vi "Write configuration to device.vi"(2 "error in (no error)":errorcluster, 3 "FP ref in":T1) -> (0 "error out":errorcluster)   [LabVIEW 2020]
uses:
  Typedefs/Front Panel Object References.ctl
  Typedefs/SDCP - Serial Port Control - Commands.ctl
  Typedefs/SDCP - Standard Message Frames FGV - Commands.ctl
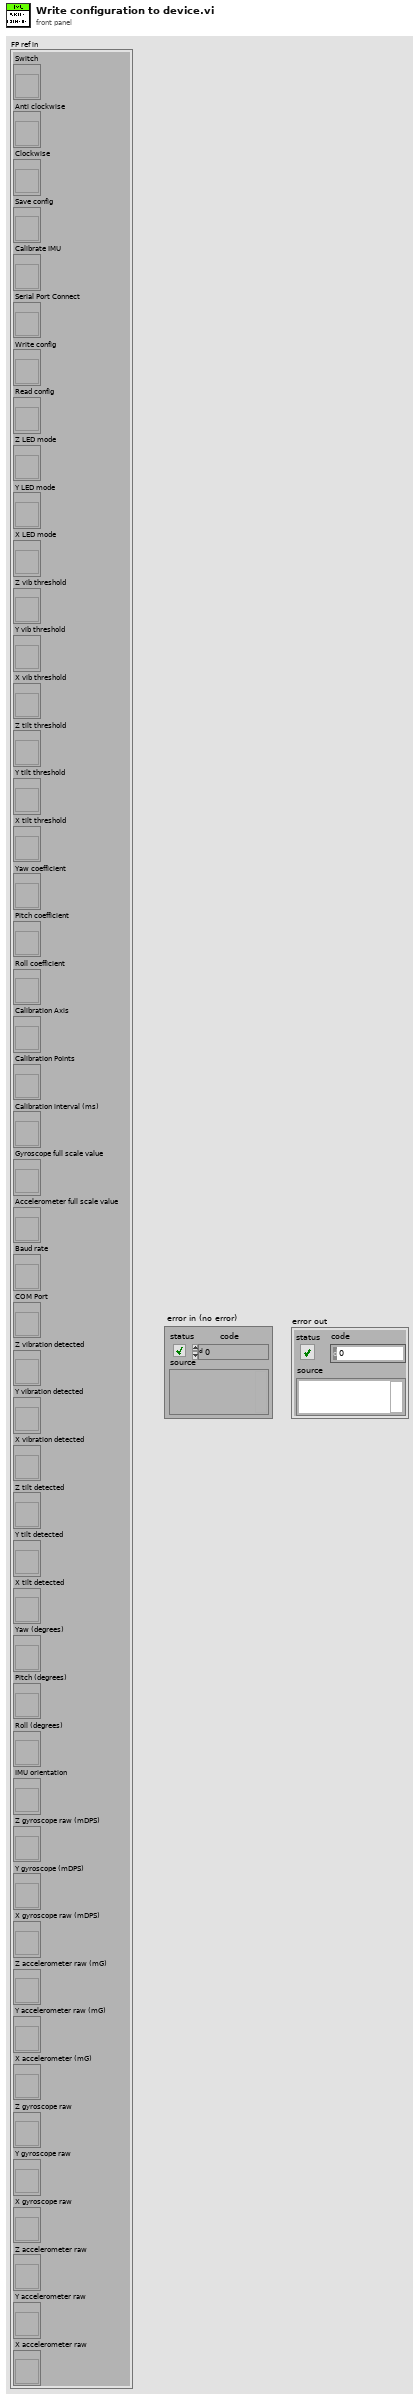
[diagram p1: front panel]
types:
  T1 = typedef "Front Panel Object References.ctl" = cluster{"Switch":refnum<vi>, "Anti clockwise":refnum<vi>, "Clockwise":refnum<vi>, "Save config":refnum<vi>, "Calibrate IMU":refnum<vi>, "Serial Port Connect":refnum<vi>, "Write config":refnum<vi>, "Read config":refnum<vi>, "Z LED mode":refnum<vi>, "Y LED mode":refnum<vi>, "X LED mode":refnum<vi>, "Z vib threshold":refnum<vi>, "Y vib threshold":refnum<vi>, "X vib threshold":refnum<vi>, "Z tilt threshold":refnum<vi>, "Y tilt threshold":refnum<vi>, "X tilt threshold":refnum<vi>, "Yaw coefficient":refnum<vi>, "Pitch coefficient":refnum<vi>, "Roll coefficient":refnum<vi>, "Calibration Axis":refnum<vi>, "Calibration Points":refnum<vi>, "Calibration interval (ms)":refnum<vi>, "Gyroscope full scale value":refnum<vi>, "Accelerometer full scale value":refnum<vi>, "Baud rate":refnum<vi>, "COM Port":refnum<vi>, "Z vibration detected":refnum<vi>, "Y vibration detected":refnum<vi>, "X vibration detected":refnum<vi>, "Z tilt detected":refnum<vi>, "Y tilt detected":refnum<vi>, "X tilt detected":refnum<vi>, "Yaw (degrees)":refnum<vi>, "Pitch (degrees)":refnum<vi>, "Roll (degrees)":refnum<vi>, "IMU orientation":refnum<vi>, "Z gyroscope raw (mDPS)":refnum<vi>, "Y gyroscope (mDPS)":refnum<vi>, "X gyroscope raw (mDPS)":refnum<vi>, "Z accelerometer raw (mG)":refnum<vi>, "Y accelerometer raw (mG)":refnum<vi>, "X accelerometer (mG)":refnum<vi>, "Z gyroscope raw":refnum<vi>, "Y gyroscope raw":refnum<vi>, "X gyroscope raw":refnum<vi>, "Z accelerometer raw":refnum<vi>, "Y accelerometer raw":refnum<vi>, "X accelerometer raw":refnum<vi>}
  T2 = typedef "SDCP - Serial Port Control - Commands.ctl" = enum16{"Open", "Read", "Write", "Get instance", "Close"}
  T3 = enum16{"X positive", "X neagtive", "Y positive", "Y negative", "Z positive", "Z negative"}
  T4 = typedef "LED mode.ctl" = enum16{"Tilt detection", "Vibration detection", "Accelerometer magnitude", "Gyroscope magnitude", "GPIO test", "PWM test"}
  T5 = typedef "SDCP - Standard Message Frames FGV - Commands.ctl" = enum16{"Reset", "Read", "Write", "Set Priority"}
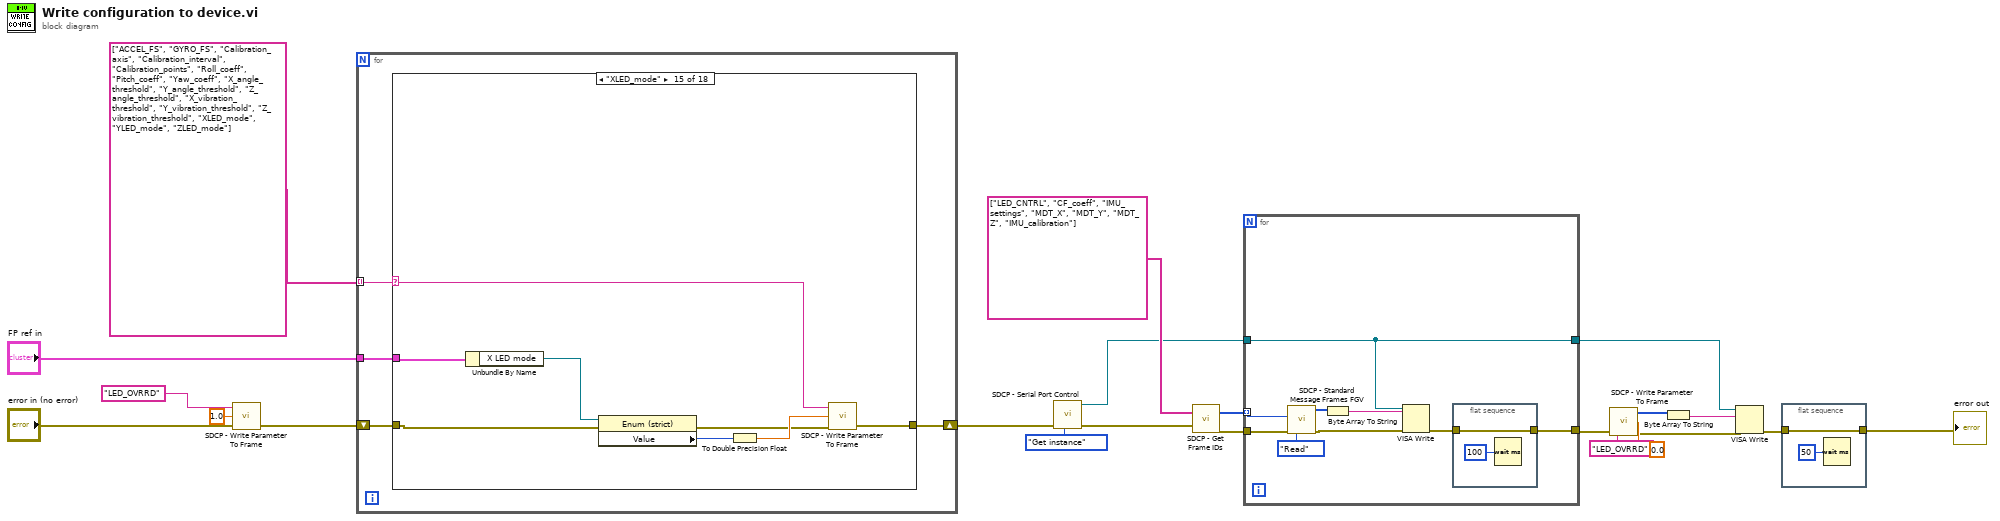
[diagram p0: block diagram]
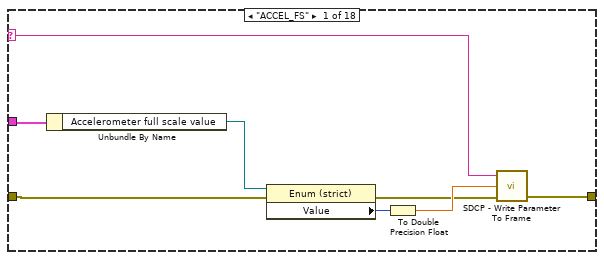
[diagram p2: hidden frame]
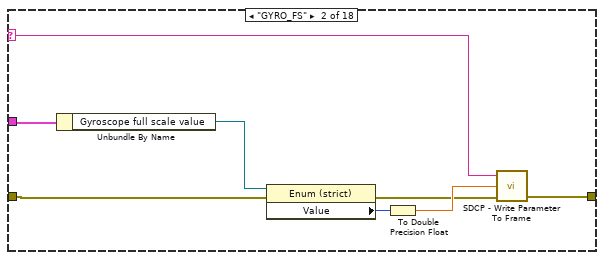
[diagram p3: hidden frame]
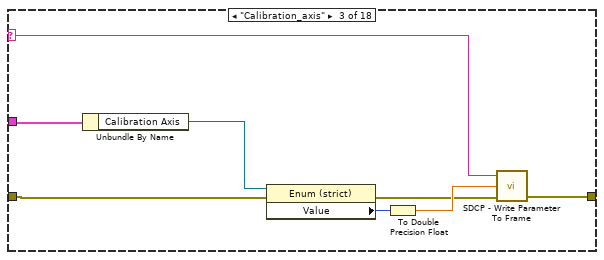
[diagram p4: hidden frame]
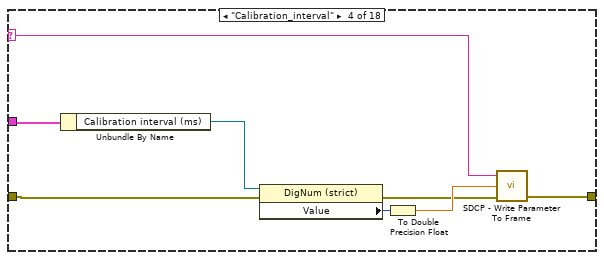
[diagram p5: hidden frame]
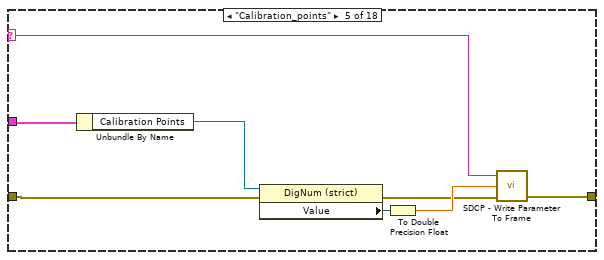
[diagram p6: hidden frame]
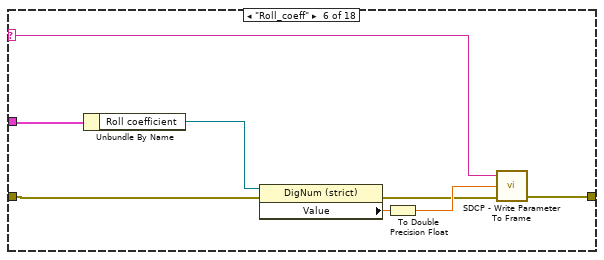
[diagram p7: hidden frame]
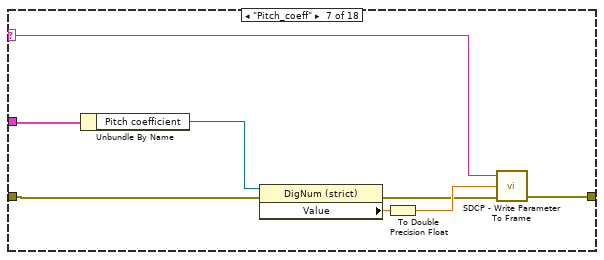
[diagram p8: hidden frame]
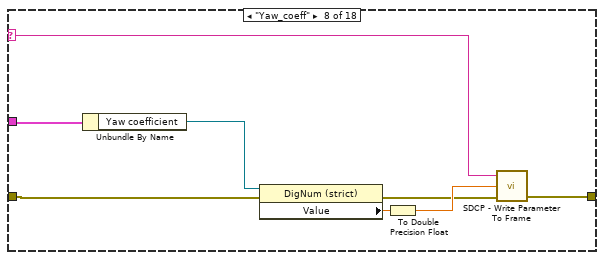
[diagram p9: hidden frame]
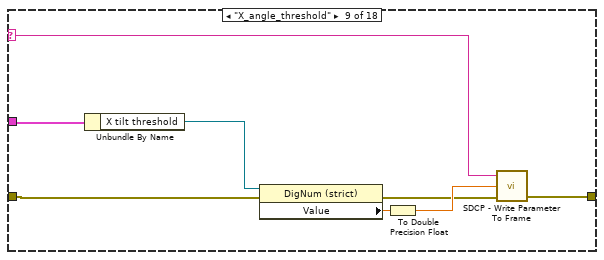
[diagram p10: hidden frame]
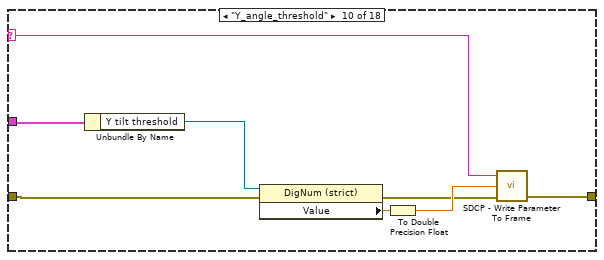
[diagram p11: hidden frame]
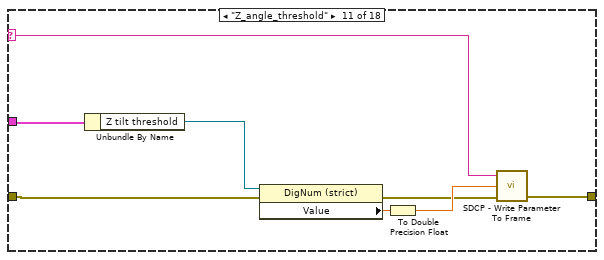
[diagram p12: hidden frame]
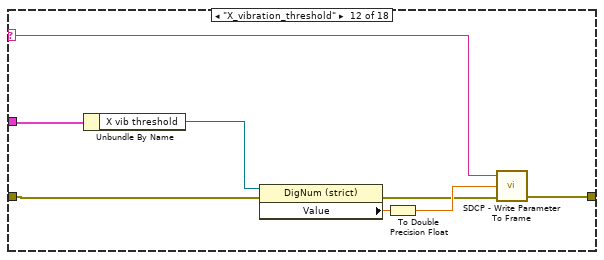
[diagram p13: hidden frame]
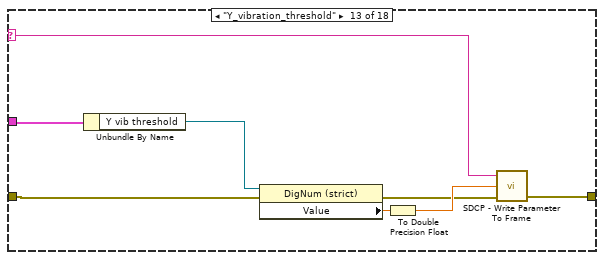
[diagram p14: hidden frame]
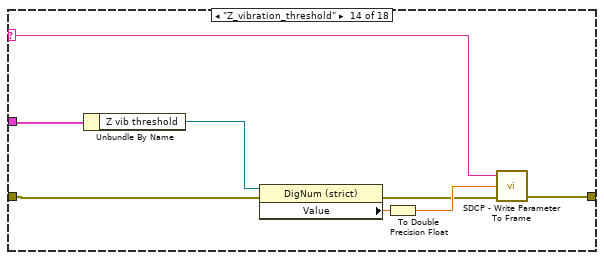
[diagram p15: hidden frame]
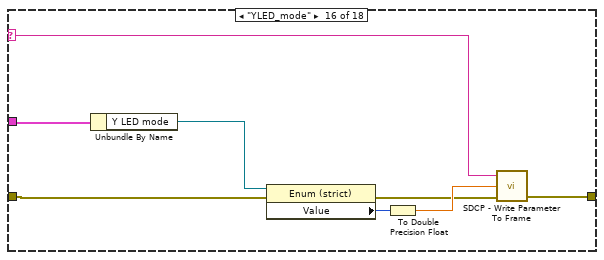
[diagram p16: hidden frame]
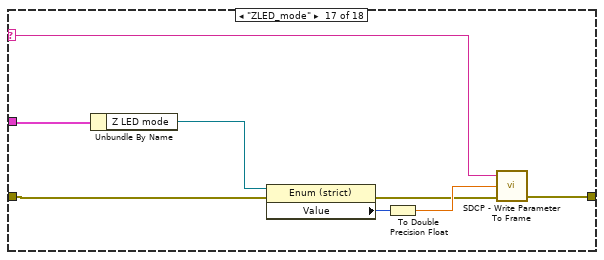
[diagram p17: hidden frame]
diagram:
  n1 = call "SDCP - Write Parameter To Frame.vi"("error in (no error)"="error in (no error)", "Value"=1.0, "Parameter Name"="LED_OVRRD") -> ("error out"=w12:errorcluster)  [unwired: 1 in, 1 out]
  n2 = for {
    tunnel: string[] ["ACCEL_FS", "GYRO_FS", "Calibration_axis", "Calibration_interval", "Calibration_points", "Roll_coeff", "Pitch_coeff", "Yaw_coeff", "X_angle_threshold", "Y_angle_threshold", "Z_angle_threshold", "X_vibration_threshold", "Y_vibration_threshold", "Z_vibration_threshold", "XLED_mode", "YLED_mode", "ZLED_mode"] -> [w26] mode=indexing
    shift-right: [w23] -> w17
    shift-left: w12 -> [w25]
    tunnel: "FP ref in" -> [w24]
    n3 = case shown="\"XLED_mode\"" w26 {
      selector: w26 -> [w33 w41 w49 w57 w65 w73 w81 w89 w97 w105 w113 w121 w129 w137 w145 w153 w161 _]
      tunnel: w25 -> [w31 w39 w47 w55 w63 w71 w79 w87 w95 w103 w111 w119 w127 w135 w143 w151 w159 w163]
      tunnel: w24 -> [w34 w42 w50 w58 w66 w74 w82 w90 w98 w106 w114 w122 w130 w138 w146 w154 w162 _]
      tunnel: [w32 w40 w48 w56 w64 w72 w80 w88 w96 w104 w112 w120 w128 w136 w144 w152 w160 w163] -> w23
      frame "ACCEL_FS" {
        n4 = Unbundle By Name(w34) -> ("Accelerometer full scale value"=w30:refnum<vi>)
        n5 = property class="Enum (strict)"(reference=w30, error in=w31) -> (error out=w27:errorcluster, "Value"=w29:enum16{"2G", "4G", "8G", "16G"})  [unwired: 1 out]
        n6 = To Double Precision Float(number=w29) -> (double precision float=w28:dbl)
        n7 = call "SDCP - Write Parameter To Frame.vi"("error in (no error)"=w27, "Value"=w28, "Parameter Name"=w33) -> ("error out"=w32:errorcluster)  [unwired: 1 in, 1 out]
      }
      frame "GYRO_FS" {
        n8 = Unbundle By Name(w42) -> ("Gyroscope full scale value"=w38:refnum<vi>)
        n9 = property class="Enum (strict)"(reference=w38, error in=w39) -> (error out=w35:errorcluster, "Value"=w37:enum16{"250DPS", "500DPS", "1000DPS", "2000DPS"})  [unwired: 1 out]
        n10 = To Double Precision Float(number=w37) -> (double precision float=w36:dbl)
        n11 = call "SDCP - Write Parameter To Frame.vi"("error in (no error)"=w35, "Value"=w36, "Parameter Name"=w41) -> ("error out"=w40:errorcluster)  [unwired: 1 in, 1 out]
      }
      frame "Calibration_axis" {
        n12 = Unbundle By Name(w50) -> ("Calibration Axis"=w46:refnum<vi>)
        n13 = property class="Enum (strict)"(reference=w46, error in=w47) -> (error out=w43:errorcluster, "Value"=w45:T3)  [unwired: 1 out]
        n14 = To Double Precision Float(number=w45) -> (double precision float=w44:dbl)
        n15 = call "SDCP - Write Parameter To Frame.vi"("error in (no error)"=w43, "Value"=w44, "Parameter Name"=w49) -> ("error out"=w48:errorcluster)  [unwired: 1 in, 1 out]
      }
      frame "Calibration_interval" {
        n16 = Unbundle By Name(w58) -> ("Calibration interval (ms)"=w54:refnum<vi>)
        n17 = property class="DigNum (strict)"(reference=w54, error in=w55) -> (error out=w51:errorcluster, "Value"=w53:u8)  [unwired: 1 out]
        n18 = To Double Precision Float(number=w53) -> (double precision float=w52:dbl)
        n19 = call "SDCP - Write Parameter To Frame.vi"("error in (no error)"=w51, "Value"=w52, "Parameter Name"=w57) -> ("error out"=w56:errorcluster)  [unwired: 1 in, 1 out]
      }
      frame "Calibration_points" {
        n20 = Unbundle By Name(w66) -> ("Calibration Points"=w62:refnum<vi>)
        n21 = property class="DigNum (strict)"(reference=w62, error in=w63) -> (error out=w59:errorcluster, "Value"=w61:u8)  [unwired: 1 out]
        n22 = To Double Precision Float(number=w61) -> (double precision float=w60:dbl)
        n23 = call "SDCP - Write Parameter To Frame.vi"("error in (no error)"=w59, "Value"=w60, "Parameter Name"=w65) -> ("error out"=w64:errorcluster)  [unwired: 1 in, 1 out]
      }
      frame "Roll_coeff" {
        n24 = Unbundle By Name(w74) -> ("Roll coefficient"=w70:refnum<vi>)
        n25 = property class="DigNum (strict)"(reference=w70, error in=w71) -> (error out=w67:errorcluster, "Value"=w69:dbl)  [unwired: 1 out]
        n26 = To Double Precision Float(number=w69) -> (double precision float=w68:dbl)
        n27 = call "SDCP - Write Parameter To Frame.vi"("error in (no error)"=w67, "Value"=w68, "Parameter Name"=w73) -> ("error out"=w72:errorcluster)  [unwired: 1 in, 1 out]
      }
      frame "Pitch_coeff" {
        n28 = Unbundle By Name(w82) -> ("Pitch coefficient"=w78:refnum<vi>)
        n29 = property class="DigNum (strict)"(reference=w78, error in=w79) -> (error out=w75:errorcluster, "Value"=w77:dbl)  [unwired: 1 out]
        n30 = To Double Precision Float(number=w77) -> (double precision float=w76:dbl)
        n31 = call "SDCP - Write Parameter To Frame.vi"("error in (no error)"=w75, "Value"=w76, "Parameter Name"=w81) -> ("error out"=w80:errorcluster)  [unwired: 1 in, 1 out]
      }
      frame "Yaw_coeff" {
        n32 = Unbundle By Name(w90) -> ("Yaw coefficient"=w86:refnum<vi>)
        n33 = property class="DigNum (strict)"(reference=w86, error in=w87) -> (error out=w83:errorcluster, "Value"=w85:dbl)  [unwired: 1 out]
        n34 = To Double Precision Float(number=w85) -> (double precision float=w84:dbl)
        n35 = call "SDCP - Write Parameter To Frame.vi"("error in (no error)"=w83, "Value"=w84, "Parameter Name"=w89) -> ("error out"=w88:errorcluster)  [unwired: 1 in, 1 out]
      }
      frame "X_angle_threshold" {
        n36 = Unbundle By Name(w98) -> ("X tilt threshold"=w94:refnum<vi>)
        n37 = property class="DigNum (strict)"(reference=w94, error in=w95) -> (error out=w91:errorcluster, "Value"=w93:dbl)  [unwired: 1 out]
        n38 = To Double Precision Float(number=w93) -> (double precision float=w92:dbl)
        n39 = call "SDCP - Write Parameter To Frame.vi"("error in (no error)"=w91, "Value"=w92, "Parameter Name"=w97) -> ("error out"=w96:errorcluster)  [unwired: 1 in, 1 out]
      }
      frame "Y_angle_threshold" {
        n40 = Unbundle By Name(w106) -> ("Y tilt threshold"=w102:refnum<vi>)
        n41 = property class="DigNum (strict)"(reference=w102, error in=w103) -> (error out=w99:errorcluster, "Value"=w101:dbl)  [unwired: 1 out]
        n42 = To Double Precision Float(number=w101) -> (double precision float=w100:dbl)
        n43 = call "SDCP - Write Parameter To Frame.vi"("error in (no error)"=w99, "Value"=w100, "Parameter Name"=w105) -> ("error out"=w104:errorcluster)  [unwired: 1 in, 1 out]
      }
      frame "Z_angle_threshold" {
        n44 = Unbundle By Name(w114) -> ("Z tilt threshold"=w110:refnum<vi>)
        n45 = property class="DigNum (strict)"(reference=w110, error in=w111) -> (error out=w107:errorcluster, "Value"=w109:dbl)  [unwired: 1 out]
        n46 = To Double Precision Float(number=w109) -> (double precision float=w108:dbl)
        n47 = call "SDCP - Write Parameter To Frame.vi"("error in (no error)"=w107, "Value"=w108, "Parameter Name"=w113) -> ("error out"=w112:errorcluster)  [unwired: 1 in, 1 out]
      }
      frame "X_vibration_threshold" {
        n48 = Unbundle By Name(w122) -> ("X vib threshold"=w118:refnum<vi>)
        n49 = property class="DigNum (strict)"(reference=w118, error in=w119) -> (error out=w115:errorcluster, "Value"=w117:dbl)  [unwired: 1 out]
        n50 = To Double Precision Float(number=w117) -> (double precision float=w116:dbl)
        n51 = call "SDCP - Write Parameter To Frame.vi"("error in (no error)"=w115, "Value"=w116, "Parameter Name"=w121) -> ("error out"=w120:errorcluster)  [unwired: 1 in, 1 out]
      }
      frame "Y_vibration_threshold" {
        n52 = Unbundle By Name(w130) -> ("Y vib threshold"=w126:refnum<vi>)
        n53 = property class="DigNum (strict)"(reference=w126, error in=w127) -> (error out=w123:errorcluster, "Value"=w125:dbl)  [unwired: 1 out]
        n54 = To Double Precision Float(number=w125) -> (double precision float=w124:dbl)
        n55 = call "SDCP - Write Parameter To Frame.vi"("error in (no error)"=w123, "Value"=w124, "Parameter Name"=w129) -> ("error out"=w128:errorcluster)  [unwired: 1 in, 1 out]
      }
      frame "Z_vibration_threshold" {
        n56 = Unbundle By Name(w138) -> ("Z vib threshold"=w134:refnum<vi>)
        n57 = property class="DigNum (strict)"(reference=w134, error in=w135) -> (error out=w131:errorcluster, "Value"=w133:dbl)  [unwired: 1 out]
        n58 = To Double Precision Float(number=w133) -> (double precision float=w132:dbl)
        n59 = call "SDCP - Write Parameter To Frame.vi"("error in (no error)"=w131, "Value"=w132, "Parameter Name"=w137) -> ("error out"=w136:errorcluster)  [unwired: 1 in, 1 out]
      }
      frame "XLED_mode" {
        n60 = Unbundle By Name(w146) -> ("X LED mode"=w142:refnum<vi>)
        n61 = property class="Enum (strict)"(reference=w142, error in=w143) -> (error out=w139:errorcluster, "Value"=w141:T4)  [unwired: 1 out]
        n62 = To Double Precision Float(number=w141) -> (double precision float=w140:dbl)
        n63 = call "SDCP - Write Parameter To Frame.vi"("error in (no error)"=w139, "Value"=w140, "Parameter Name"=w145) -> ("error out"=w144:errorcluster)  [unwired: 1 in, 1 out]
      }
      frame "YLED_mode" {
        n64 = Unbundle By Name(w154) -> ("Y LED mode"=w150:refnum<vi>)
        n65 = property class="Enum (strict)"(reference=w150, error in=w151) -> (error out=w147:errorcluster, "Value"=w149:T4)  [unwired: 1 out]
        n66 = To Double Precision Float(number=w149) -> (double precision float=w148:dbl)
        n67 = call "SDCP - Write Parameter To Frame.vi"("error in (no error)"=w147, "Value"=w148, "Parameter Name"=w153) -> ("error out"=w152:errorcluster)  [unwired: 1 in, 1 out]
      }
      frame "ZLED_mode" {
        n68 = Unbundle By Name(w162) -> ("Z LED mode"=w158:refnum<vi>)
        n69 = property class="Enum (strict)"(reference=w158, error in=w159) -> (error out=w155:errorcluster, "Value"=w157:T4)  [unwired: 1 out]
        n70 = To Double Precision Float(number=w157) -> (double precision float=w156:dbl)
        n71 = call "SDCP - Write Parameter To Frame.vi"("error in (no error)"=w155, "Value"=w156, "Parameter Name"=w161) -> ("error out"=w160:errorcluster)  [unwired: 1 in, 1 out]
      }
      frame Default {
      }
    }
  }
  n72 = call "SDCP - Serial Port Control.vi"("Command"=SDCP_-_Serial_Port_Control_-_Commands."Get instance", "error in (no error)"=w17) -> ("error out"=w16:errorcluster, "VISA out"=w14:refnum<visa-resource-name>)  [unwired: 6 in, 2 out]
  n73 = call "SDCP - Get Frame IDs.vi"("error in (no error)"=w16, "Frame names"=string[] ["LED_CNTRL", "CF_coeff", "IMU_settings", "MDT_X", "MDT_Y", "MDT_Z", "IMU_calibration"]) -> ("error out"=w19:errorcluster, "Frame IDs"=w18:u8[])
  n74 = for {
    tunnel: w19 -> [w172]
    tunnel: w18 -> [w170] mode=indexing
    tunnel: w14 -> [w164]
    tunnel: [w165] -> w9
    tunnel: [w164] -> w5
    n75 = call "SDCP - Standard Message Frames FGV.vi"("error in (no error)"=w172, "Command"=SDCP_-_Standard_Message_Frames_FGV_-_Commands."Read", "FID"=w170) -> ("error out"=w169:errorcluster, "SMF out"=w168:u8[])  [unwired: 3 in, 1 out]
    n76 = Byte Array To String(unsigned byte array=w168) -> (string=w167:string)
    n77 = VISA Write(VISA resource name=w164, write buffer=w167, error in (no error)=w169) -> (error out=w166:errorcluster)  [unwired: 2 out]
    n78 = flat-sequence {
      tunnel: w166 -> [w174]
      tunnel: [w174] -> w165
      frame #0 {
        n79 = Wait (ms)(milliseconds to wait=u32 100) -> ()  [unwired: 1 out]
      }
    }
  }
  n80 = call "SDCP - Write Parameter To Frame.vi"("error in (no error)"=w9, "Value"=0.0, "Parameter Name"="LED_OVRRD") -> ("error out"=w6:errorcluster, "Encoded message frame"=w4:u8[])  [unwired: 1 in]
  n81 = Byte Array To String(unsigned byte array=w4) -> (string=w3:string)
  n82 = VISA Write(VISA resource name=w5, write buffer=w3, error in (no error)=w6) -> (error out=w2:errorcluster)  [unwired: 2 out]
  n83 = flat-sequence {
    tunnel: w2 -> [w176]
    tunnel: [w176] -> w1
    frame #0 {
      n84 = Wait (ms)(milliseconds to wait=u32 50) -> ()  [unwired: 1 out]
    }
  }
  "error out" <- w1
